vi "PNA_Set Marker Position.vi"(0 "VISA resource name":refnum<visa-resource-name>, 1 "Channel (1)":i32=1, 2 "Trace (1)":i32=1, 3 "Marker (1)":i32=1, 5 "X Value (0.0)":dbl format="%.6f", 11 "error in (no error)":errorcluster, 12 "Units":enum16{"Hz", "MHz", "GHz"}(ring)) -> (4 "VISA resource name out":refnum<visa-resource-name>, 15 "error out":errorcluster)   [LabVIEW 2018, in "Agilent ENA Series.lvlib"]
doc: "Sets the marker location."
uses:
  Agilent ENA Series.lvlib
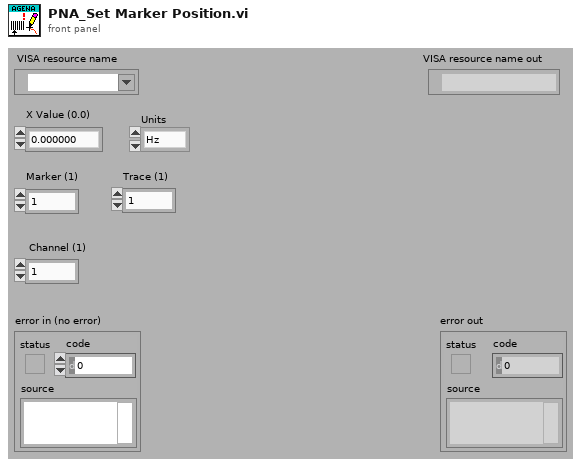
[diagram p1: front panel]
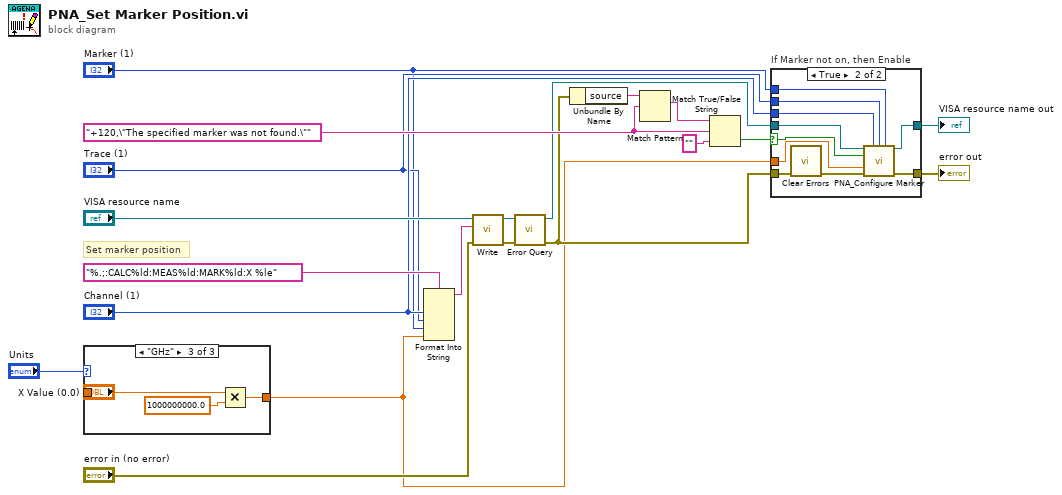
[diagram p0: block diagram]
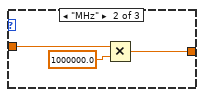
[diagram p4: hidden frame]
diagram:
  w12 = "+120,\"The specified marker was not found.\"" ("regular expression")
  # "Set marker position"
  n1 = case shown="\"GHz\"" "Units" {
    tunnel: "X Value (0.0)" -> [w22 w25 w28]
    tunnel: [w22 w23 w26] -> w2
    frame "Hz", Default {
    }
    frame "MHz" {
      n2 = Multiply(x=w25, y=1000000.0) -> (x*y=w23:dbl)
    }
    frame "GHz" {
      n3 = Multiply(x=w28, y=1000000000.0) -> (x*y=w26:dbl)
    }
  }
  n4 = Format Into String(format string="%.;:CALC%ld:MEAS%ld:MARK%ld:X %le", "Channel (1)", "Trace (1)", "Marker (1)", w2) -> (resulting string=w19:string)  [unwired: 2 in, 1 out]
  n5 = call "Write.vi"("error in (no error)"="error in (no error)", "String ()"=w19, "VISA resource name"="VISA resource name") -> ("error out"=w17:errorcluster, "VISA resource name out"=w18:refnum<visa-resource-name>)  [unwired: 6 in, 1 out]
  n6 = call "Error Query.vi"("error in (no error)"=w17, "VISA resource name"=w18) -> ("error out"=w3:errorcluster, "VISA resource name out"=w8:refnum<visa-resource-name>)  [unwired: 6 in, 2 out]
  n7 = Unbundle By Name(w3) -> ("source"=w13:string)
  n8 = Match Pattern(string=w13, regular expression=w12) -> (match substring=w10:string)  [unwired: 1 in, 3 out]
  n9 = Match True/False String(2:"" ("false string"), 3:w12, 4:w10) -> (0:w9:bool)  [unwired: 1 out]
  n10 = case "If Marker not on, then Enable" shown="True" w9 {
    selector: w9 -> [_ w34]
    tunnel: w8 -> [w30 w40]
    tunnel: [w30 w39] -> w7
    tunnel: "Channel (1)" -> [_ w38]
    tunnel: "Trace (1)" -> [_ w37]
    tunnel: "Marker (1)" -> [_ w36]
    tunnel: w3 -> [w29 w31]
    tunnel: w2 -> [_ w35]
    tunnel: [w29 w33] -> w1
    frame False {
    }
    frame True {
      n11 = call <vilib>:"Clear Errors.vi"("error in (no error)"=w31) -> ("error out"=w32:errorcluster)  [unwired: 5 in, 1 out]
      n12 = call "PNA_Configure Marker.vi"("VISA resource name"=w40, "Channel (1)"=w38, "Trace (1)"=w37, "Marker (1)"=w36, "Marker State (F: Disabled)"=w34, "Mkr Freq"=w35, "error in (no error)"=w32) -> ("VISA resource name out"=w39:refnum<visa-resource-name>, "error out"=w33:errorcluster)  [unwired: 7 in]
    }
  }
  "error out" <- w1
  "VISA resource name out" <- w7
